vi "StateMachineTest2.vi"() -> ()   [LabVIEW 2019]
uses:
  StateMachineTest2_State.vi
  <vilib>/Utility/miscctls.llb/LVPositionTypeDef.ctl
panel:
  out "State":T1
  in  "Start":bool
  out "Ball2":bool
  out "Ball1":bool
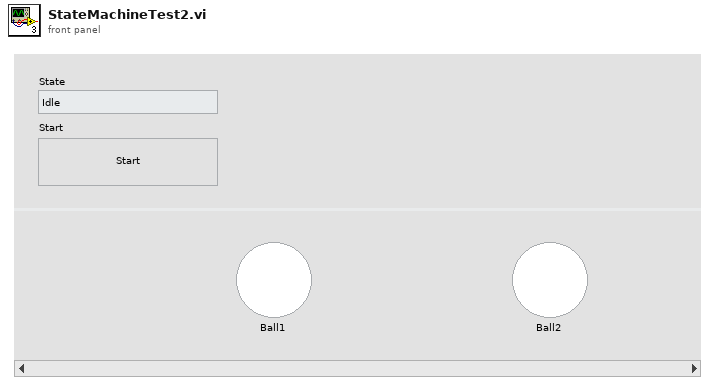
[diagram p1: front panel]
types:
  T1 = typedef "StateMachineTest2_State.vi" = enum16{"Idle", "Initialize", "Ball1 move to Ball2", "Ball2 blink", "Ball2 move a little"}
  T2 = typedef "LVPositionTypeDef.ctl" = cluster{"Left":i32, "Top":i32}
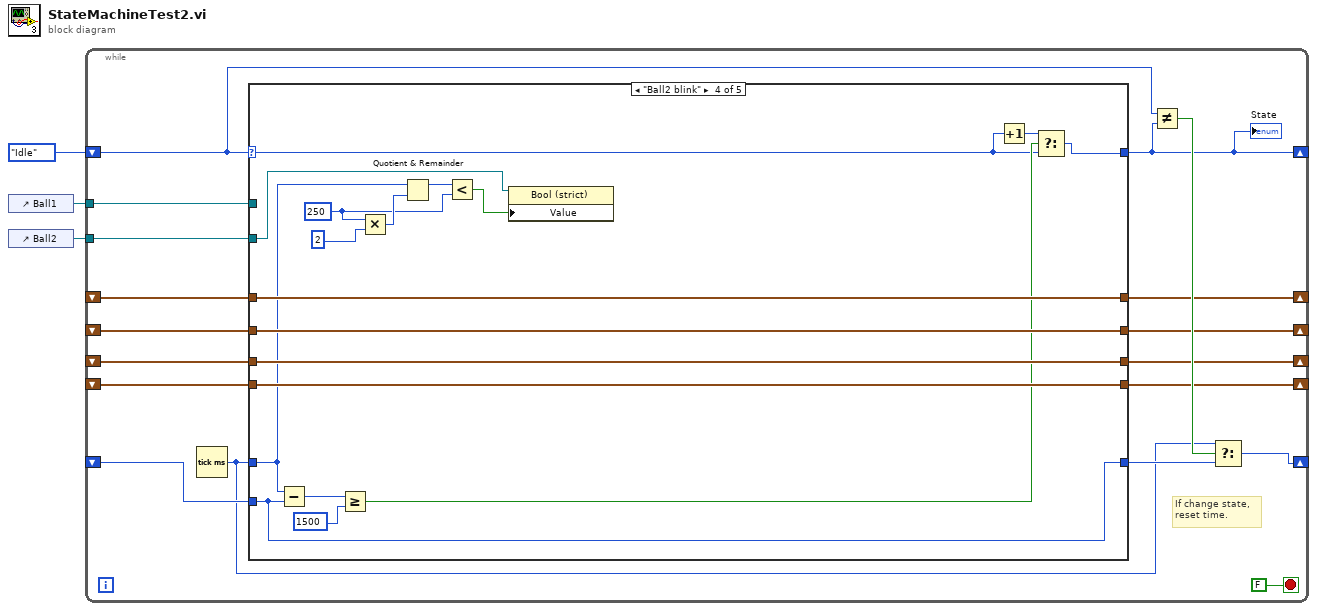
[diagram p0: block diagram]
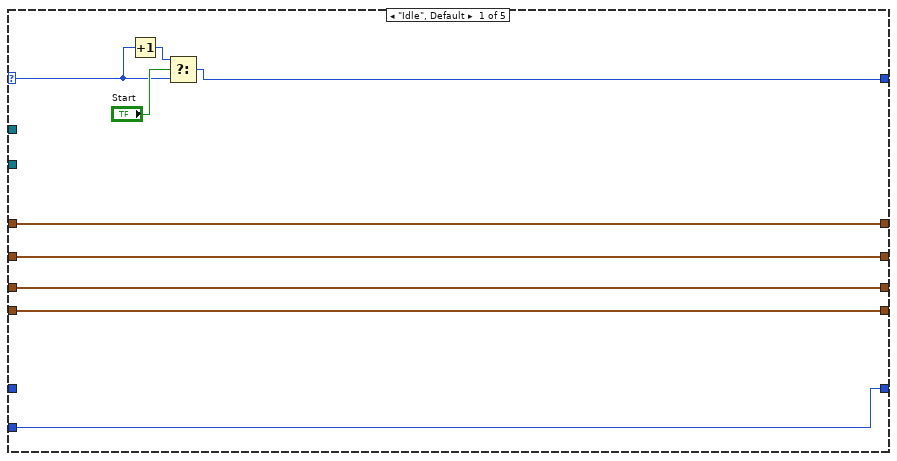
[diagram p2: hidden frame]
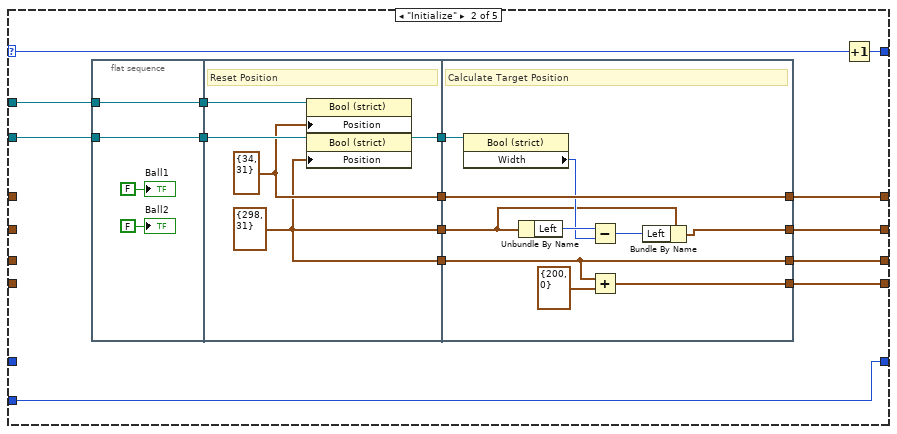
[diagram p3: hidden frame]
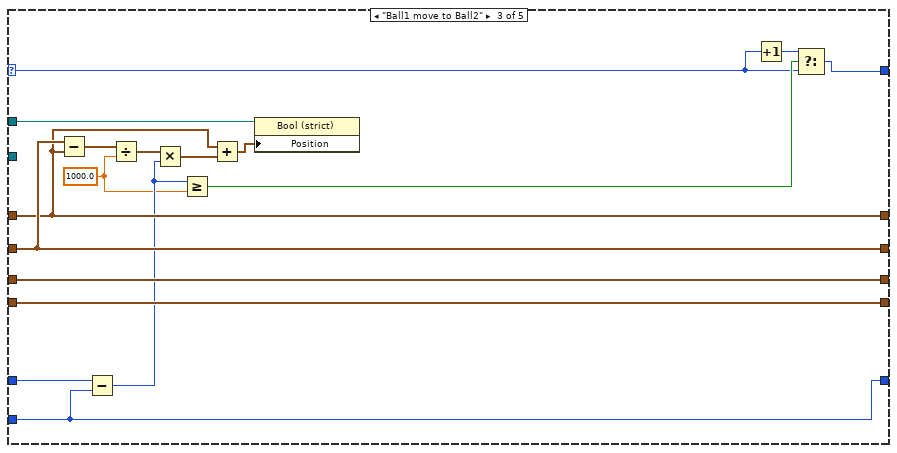
[diagram p4: hidden frame]
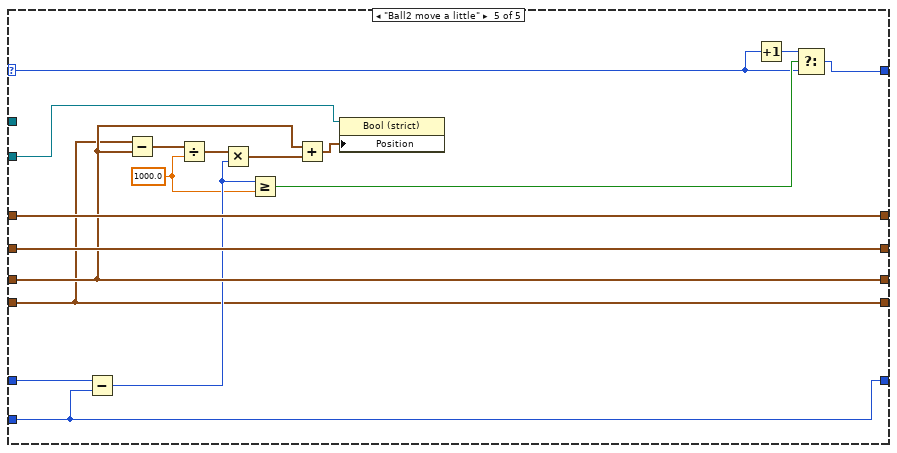
[diagram p5: hidden frame]
diagram:
  n1 = control-ref of="Ball1"() -> (w2:refnum<vi>)
  n2 = control-ref of="Ball2"() -> (w1:refnum<vi>)
  n3 = while {
    shift-right: [w12] -> _
    shift-left: StateMachineTest2_State.vi."Idle" -> [w11]
    tunnel: w2 -> [w19]
    tunnel: w1 -> [w18]
    shift-right: [w16] -> _
    shift-left: _ -> [w14]
    shift-right: [w17] -> _
    shift-left: _ -> [w15]
    shift-right: [w9] -> _
    shift-left: _ -> [w13]
    shift-right: [w7] -> _
    shift-left: _ -> [w6]
    shift-right: [w5] -> _
    shift-left: _ -> [w4]
    stop <- FALSE stop-if-true
    # "If change state,\nreset time."
    n4 = Tick Count (ms)() -> (millisecond timer value=w8:u32)
    n5 = case shown="\"Ball2 blink\"" w11 {
      selector: w11 -> [w27 w41 w65 w82 w103]
      tunnel: [w30 w40 w70 w97 w107] -> w12
      tunnel: w19 -> [_ w45 w77 _ _]
      tunnel: w18 -> [_ w44 _ w84 w102]
      tunnel: [w26 w43 w81 w96 w116] -> w17
      tunnel: [w25 w42 w80 w95 w115] -> w16
      tunnel: w15 -> [w26 _ w81 w96 w116]
      tunnel: w14 -> [w25 _ w80 w95 w115]
      tunnel: [w24 w36 w74 w85 w111] -> w10
      tunnel: w8 -> [_ _ w75 w89 w112]
      tunnel: w13 -> [w24 w36 w74 w85 w111]
      tunnel: [w23 w35 w79 w98 w114] -> w7
      tunnel: w6 -> [w23 _ w79 w98 w114]
      tunnel: [w22 w33 w78 w99 w100] -> w5
      tunnel: w4 -> [w22 _ w78 w99 w100]
      frame "Idle", Default {
        n6 = Increment(x=w27) -> (x+1=w28:T1)
        n7 = Select(t=w28, s="Start", f=w27) -> (s? t:f=w30:T1)
      }
      frame "Initialize" {
        n8 = flat-sequence {
          tunnel: w44 -> [w48]
          tunnel: w45 -> [w49]
          tunnel: [w49] -> w32
          tunnel: [w48] -> w31
          tunnel: [w50] -> w39
          tunnel: [w52] -> w38
          tunnel: [w51] -> w37
          tunnel: [w50] -> w34
          tunnel: w32 -> [w54]
          tunnel: w31 -> [w53]
          tunnel: [w64] -> w42
          tunnel: [w58] -> w43
          tunnel: w39 -> [w60]
          tunnel: w38 -> [w64]
          tunnel: w37 -> [w63]
          tunnel: [w57] -> w35
          tunnel: w34 -> [w57]
          tunnel: [w55] -> w33
          frame #0 {
            "Ball1" <- FALSE ("Ball1")
            "Ball2" <- FALSE ("Ball2")
          }
          frame #1 {
            w50 = T2 {"Left"=298, "Top"=31} ("Position 2")
            w52 = T2 {"Left"=34, "Top"=31} ("Position")
            # "Reset Position"
            n9 = property class="Bool (strict)"(reference=w54, "Position"=w52) -> ()  [unwired: 1 in, 2 out]
            n10 = property class="Bool (strict)"(reference=w53, "Position"=w50) -> (reference out=w51:refnum<vi>)  [unwired: 1 in, 1 out]
          }
          frame #2 {
            # "Calculate Target Position"
            n11 = property class="Bool (strict)"(reference=w63) -> ("Width"=w61:u32)  [unwired: 1 in, 2 out]
            n12 = Unbundle By Name(w60) -> ("Left"=w62:i32)
            n13 = Subtract(x=w62, y=w61) -> (x-y=w59:u32)
            n14 = Add(x=w57, y=T2 {"Left"=200, "Top"=0}) -> (x+y=w55:T2)
            n15 = Bundle By Name(cluster=w60, "Left"=w59) -> (w58:T2)
          }
        }
        n16 = Increment(x=w41) -> (x+1=w40:T1)
      }
      frame "Ball1 move to Ball2" {
        w71 = 1000.0
        n17 = Subtract(x=w81, y=w80) -> (x-y=w76:T2)
        n18 = Subtract(x=w75, y=w74) -> (x-y=w72:u32)
        n19 = Divide(x=w76, y=w71) -> (x/y=w73:cluster{"Left":dbl, "Top":dbl})
        n20 = Multiply(x=w73, y=w72) -> (x*y=w68:cluster{"Left":dbl, "Top":dbl})
        n21 = Greater Or Equal?(x=w72, y=w71) -> (x >= y?=w69:bool)
        n22 = Add(x=w80, y=w68) -> (x+y=w67:cluster{"Left":dbl, "Top":dbl})
        n23 = property class="Bool (strict)"(reference=w77, "Position"=w67) -> ()  [unwired: 1 in, 2 out]
        n24 = Increment(x=w65) -> (x+1=w66:T1)
        n25 = Select(t=w66, s=w69, f=w65) -> (s? t:f=w70:T1)
      }
      frame "Ball2 blink" {
        w91 = 250
        n26 = Subtract(x=w89, y=w85) -> (x-y=w88:u32)
        n27 = Greater Or Equal?(x=w88, y=u32 1500) -> (x >= y?=w86:bool)
        n28 = Multiply(x=w91, y=2) -> (x*y=w93:i32)
        n29 = Quotient & Remainder(x=w89, y=w93) -> (x-y*floor(x/y)=w92:u32)  [unwired: 1 out]
        n30 = Less?(x=w92, y=w91) -> (x < y?=w90:bool)
        n31 = property class="Bool (strict)"(reference=w84, "Value"=w90) -> ()  [unwired: 1 in, 2 out]
        n32 = Increment(x=w82) -> (x+1=w83:T1)
        n33 = Select(t=w83, s=w86, f=w82) -> (s? t:f=w97:T1)
      }
      frame "Ball2 move a little" {
        w108 = 1000.0
        n34 = Subtract(x=w112, y=w111) -> (x-y=w109:u32)
        n35 = Subtract(x=w100, y=w114) -> (x-y=w113:T2)
        n36 = Divide(x=w113, y=w108) -> (x/y=w110:cluster{"Left":dbl, "Top":dbl})
        n37 = Multiply(x=w110, y=w109) -> (x*y=w101:cluster{"Left":dbl, "Top":dbl})
        n38 = Greater Or Equal?(x=w109, y=w108) -> (x >= y?=w106:bool)
        n39 = Add(x=w114, y=w101) -> (x+y=w105:cluster{"Left":dbl, "Top":dbl})
        n40 = property class="Bool (strict)"(reference=w102, "Position"=w105) -> ()  [unwired: 1 in, 2 out]
        n41 = Increment(x=w103) -> (x+1=w104:T1)
        n42 = Select(t=w104, s=w106, f=w103) -> (s? t:f=w107:T1)
      }
    }
    "State" <- w12
    n43 = Not Equal?(x=w11, y=w12) -> (x != y?=w21:bool)
    n44 = Select(t=w8, s=w21, f=w10) -> (s? t:f=w9:u32)
  }
